vi "create.noManifest_trueFrameRate.vi"(9 "trueFrameRate":dbl, 10 "startingTimestamp":cluster{"seconds":i64, "nanos":i64, "picos":i64}) -> (3 "Timestamp Manifest":refnum<class "noManifest.lvclass">)   [LabVIEW 2020, in "nominal types.lvlib" / "timestampManifest.lvlib"]
uses:
  timestampManifest.lvlib
  noManifest/noManifest.lvclass
  trueFrameRate/trueFrameRate.lvclass
  C:/code/labview-client/lv_src/nominal types/timestampManifest/scaleParameter/scaleParameter.lvclass
  C:/code/labview-client/lv_src/Nominal Client/datasources/payload/payload.lvclass
  C:/code/labview-client/lv_src/nominal types/timestampManifest/trueFrameRate/trueFrameRate.lvclass
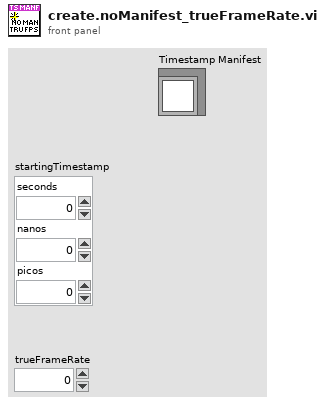
[diagram p1: front panel]
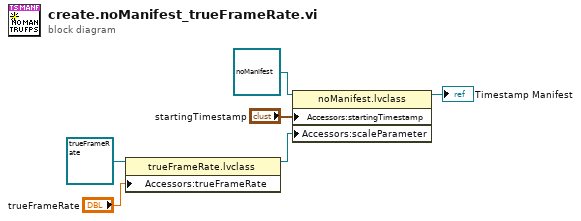
[diagram p0: block diagram]
diagram:
  n1 = property class="trueFrameRate.lvclass"(reference=refnum<class "trueFrameRate.lvclass"> refnum ("nominal types.lvlib:timestampManifest.lvlib:trueFrameRate.lvclass"), "Accessors:trueFrameRate"="trueFrameRate") -> (reference out=w3:refnum<class "trueFrameRate.lvclass">)  [unwired: 1 in, 1 out]
  n2 = property class="noManifest.lvclass"(reference=refnum<class "noManifest.lvclass"> refnum ("nominal types.lvlib:timestampManifest.lvlib:noManifest.lvclass"), "Accessors:startingTimestamp"="startingTimestamp", "Accessors:scaleParameter"=w3) -> (reference out=→"Timestamp Manifest":refnum<class "noManifest.lvclass">)  [unwired: 1 in, 1 out]
